vi "global variable.vi"() -> ()   [LabVIEW 2015]
panel:
  in  "I_Load_Inv_T":dbl
  in  "I_Load_Inv_S":dbl
  in  "I_Load_Inv_R":dbl
  in  "Vac_input3":dbl
  in  "Vac_input2":dbl
  in  "Vac_input1":dbl
  in  "Ubat":dbl
  in  "Ibat":dbl
  in  "Nivel_bat_out":dbl
  in  "Pot_load_out":dbl
  in  "Pot_panel_out":dbl
  in  "Time_inv":timestamp
  in  "Time_gen":timestamp
  in  "Pot_gen":dbl
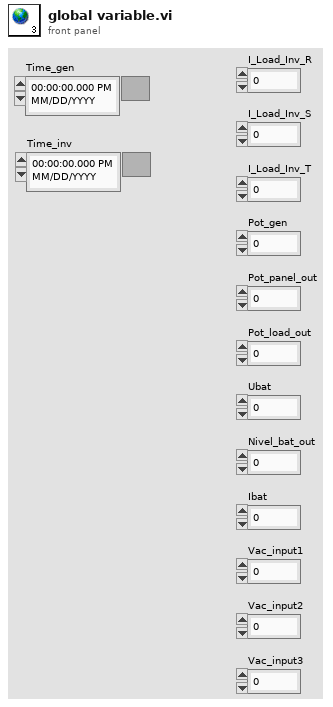
[diagram p1: front panel]
diagram:
